vi "enumerateStaticDependencies.vi"(8 "error in (no error)":errorcluster, 11 "SMO.Example":refnum<class "SMO.TopLevel.lvclass">) -> (0 "error out":errorcluster, 2 "Static Dependencies":refnum<class "Dependency.lvclass">[](array[class]), 3 "SMO.Example out":refnum<class "SMO.TopLevel.lvclass">)   [LabVIEW 2013, in "SMO.TopLevel.lvclass"]
uses:
  SMO.TopLevel.lvclass
  src/Dependency/Dependency.lvclass
  Typedefs/Dependencies--Cluster.ctl
  SMO.A/SMO.A.lvclass
  src/SMO/SMO.lvclass
panel:
  # "For instructions on how to use the JKI State Machine Objects, examples and video tutorials, visit:\nhttp://jki.net/state-machine-objects/\n\nJKI State Machine Objects™\nhttp://jki.net/state-machine-objects/\nCopyright (C) 2005-2015, JKI <info@jki.net>\nALL RIGHTS RESERVED"
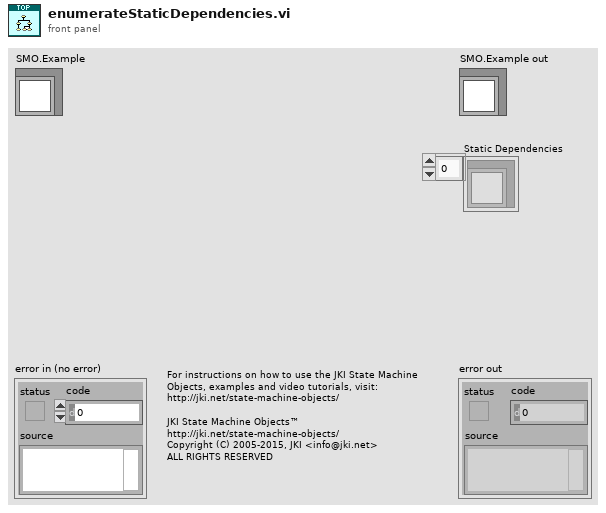
[diagram p1: front panel]
types:
  T1 = typedef "SMO.TopLevel.lvclass/Dependencies--Cluster.ctl" = cluster{"A":refnum<class "SMO.A.lvclass">}
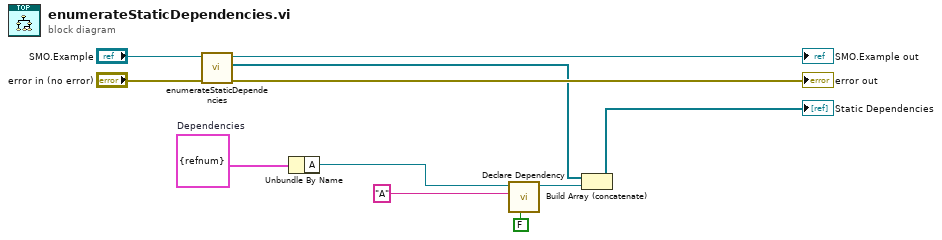
[diagram p0: block diagram]
diagram:
  w2 = T1 {"A"=refnum}  # Dependencies
  n1 = call-parent "enumerateStaticDependencies.vi"("error in (no error)"="error in (no error)", "SMO"="SMO.Example") -> ("error out"=→"error out":errorcluster, "Static Dependencies"=w3:refnum<class "Dependency.lvclass">[], "SMO out"=→"SMO.Example out":refnum<class "SMO.TopLevel.lvclass">)  [unwired: 7 in]
  n2 = Unbundle By Name(w2) -> ("A"=w1:refnum<class "SMO.A.lvclass">)
  n3 = call "Declare Dependency.vi"("Shared Resource (F)"=FALSE, "Name"="A", "Type"=w1) -> ("Dependency out"=w6:refnum<class "Dependency.lvclass">)  [unwired: 7 in, 1 out]
  n4 = Build Array (concatenate)(w3, w6) -> (→"Static Dependencies":refnum<class "Dependency.lvclass">[])
